vi "Steering Vectors.vi"(0 "rotation":dbl) -> (3 "BL Vector":cluster{dbl, dbl}, 4 "BR Vector":cluster{dbl, dbl}, 5 "FR Vector":cluster{dbl, dbl}, 6 "FL Vector":cluster{dbl, dbl})   [LabVIEW 2019]
uses:
  swerveData.vi
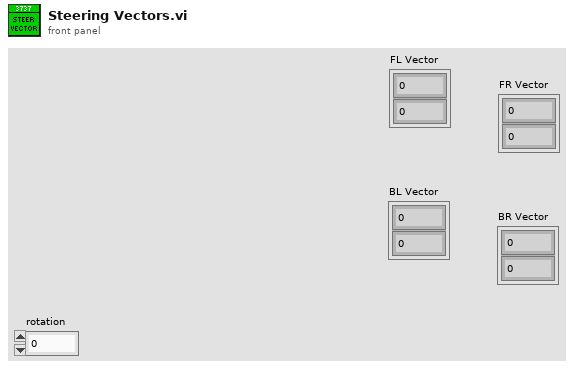
[diagram p1: front panel]
types:
  T1 = cluster{"[0]":dbl, "[1]":dbl, "[2]":dbl, "[3]":dbl, "[4]":dbl, "[5]":dbl, "[6]":dbl, "[7]":dbl, "[8]":dbl}
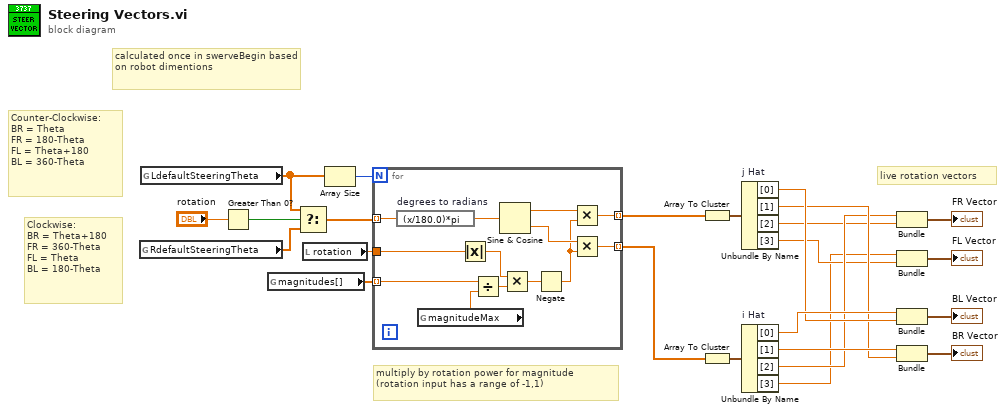
[diagram p0: block diagram]
diagram:
  # "live rotation vectors"
  # "multiply by rotation power for magnitude\n(rotation input has a range of -1,1)"
  # "calculated once in swerveBegin based on robot dimentions"
  # "Clockwise:\nBR = Theta+180\nFR = 360-Theta\nFL = Theta\nBL = 180-Theta"
  # "Counter-Clockwise:\nBR = Theta\nFR = 180-Theta\nFL = Theta+180\nBL = 360-Theta"
  n1 = global read "swerveData.vi" "RdefaultSteeringTheta"() -> (w10:dbl[])
  n2 = global read "swerveData.vi" "LdefaultSteeringTheta"() -> (w2:dbl[])
  n3 = Greater Than 0?(x="rotation") -> (x > 0?=w11:bool)
  n4 = global read "swerveData.vi" "magnitudes[]"() -> (w4:dbl[])
  n5 = Select(t=w2, s=w11, f=w10) -> (s? t:f=w9:dbl[])
  n6 = local read "rotation"() -> (w1:dbl)
  n7 = Array Size(array=w2) -> (size(s)=w3:i32)
  n8 = for {
    N: w3 -> [_]
    tunnel: [w34] -> w13 mode=indexing
    tunnel: [w33] -> w12 mode=indexing
    tunnel: w9 -> [w32] mode=indexing
    tunnel: w4 -> [w28] mode=indexing
    tunnel: w1 -> [w25]
    n9 = expression code="(x/180.0)*pi" "degrees to radians"(w32) -> (w37:dbl)
    n10 = global read "swerveData.vi" "magnitudeMax"() -> (w29:dbl)
    n11 = Absolute Value(x=w25) -> (abs(x)=w31:dbl)
    n12 = Divide(x=w28, y=w29) -> (x/y=w30:dbl)
    n13 = Sine & Cosine(0:w37) -> (1:w36:dbl, 2:w35:dbl)
    n14 = Multiply(x=w31, y=w30) -> (x*y=w27:dbl)
    n15 = Negate(x=w27) -> (-x=w26:dbl)
    n16 = Multiply(x=w36, y=w26) -> (x*y=w34:dbl)
    n17 = Multiply(x=w35, y=w26) -> (x*y=w33:dbl)
  }
  n18 = Array To Cluster(array=w13) -> (cluster=w22:T1)
  n19 = Array To Cluster(array=w12) -> (cluster=w23:T1)
  n20 = Unbundle By Name "j Hat"(w22) -> ("[0]"=w20:dbl, "[1]"=w18:dbl, "[2]"=w16:dbl, "[3]"=w15:dbl)
  n21 = Unbundle By Name "i Hat"(w23) -> ("[0]"=w21:dbl, "[1]"=w19:dbl, "[2]"=w17:dbl, "[3]"=w14:dbl)
  n22 = Bundle("[2]"=w17, "[2]"=w16) -> (→"FR Vector":cluster{"[2]":dbl, "[2]":dbl})  [unwired: 1 in]
  n23 = Bundle("[3]"=w14, "[3]"=w15) -> (→"FL Vector":cluster{"[3]":dbl, "[3]":dbl})  [unwired: 1 in]
  n24 = Bundle("[0]"=w21, "[0]"=w20) -> (→"BL Vector":cluster{"[0]":dbl, "[0]":dbl})  [unwired: 1 in]
  n25 = Bundle("[1]"=w19, "[1]"=w18) -> (→"BR Vector":cluster{"[1]":dbl, "[1]":dbl})  [unwired: 1 in]
